vi "Direct Message Sent.vi"(8 "error in (no error)":errorcluster, 10 "Message":T1, 11 "Msg Forward Interface Actor in":refnum<class "Msg Forward Interface Actor.lvclass">) -> (0 "error out":errorcluster, 3 "Msg Forward Interface Actor out":refnum<class "Msg Forward Interface Actor.lvclass">)   [LabVIEW 2020, in "Msg Forward Interface Actor.lvlib" / "Msg Forward Interface Actor.lvclass"]
uses:
  Msg Forward Interface Actor.lvclass
  Controls/Message Control.ctl
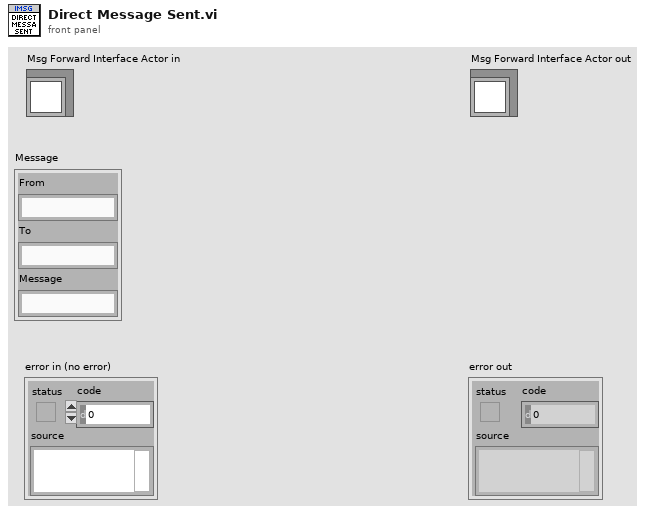
[diagram p1: front panel]
types:
  T1 = typedef "Message Control.ctl" = cluster{"From":string, "To":string, "Message":string}
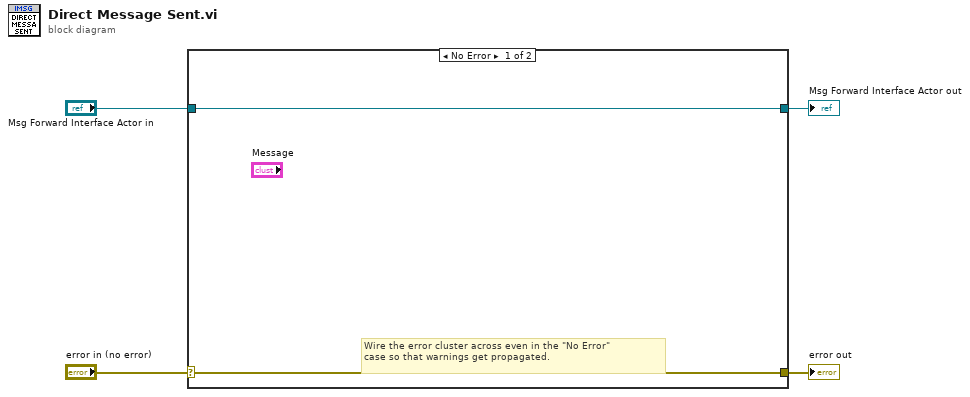
[diagram p0: block diagram]
diagram:
  n1 = case shown="No Error" "error in (no error)" {
    selector: "error in (no error)" -> [w5 w8]
    tunnel: [w5 w8] -> w3
    tunnel: [w6 w7] -> w1
    tunnel: "Msg Forward Interface Actor in" -> [w6 w7]
    frame No Error {
      # "Wire the error cluster across even in the \"No Error\"\ncase so that warnings get propagated."
    }
    frame Error {
    }
  }
  "error out" <- w3
  "Msg Forward Interface Actor out" <- w1
